vi "To CSV File.vi"(8 "error in (no error)":errorcluster, 9 "Path":path, 10 "engine configuration":refnum<class "engine configuration.lvclass">, 11 "module editor node in":refnum<class "module editor node.lvclass">) -> (0 "error out":errorcluster, 3 "module editor node out":refnum<class "module editor node.lvclass">)   [LabVIEW 2014, in "PL Framework Configuration Tool.lvlib" / "module editor node.lvclass"]
uses:
  module editor node.lvclass
  <vilib>/NI/Module Execution Interface/Engine Configuration/engine configuration.lvclass
  <vilib>/NI/Tag Bus Module Framework/module configuration/TBM module configuration.lvclass
  <vilib>/NI/Configuration Framework/serializable configuration/NISE_CEF_serializable configuration.lvclass
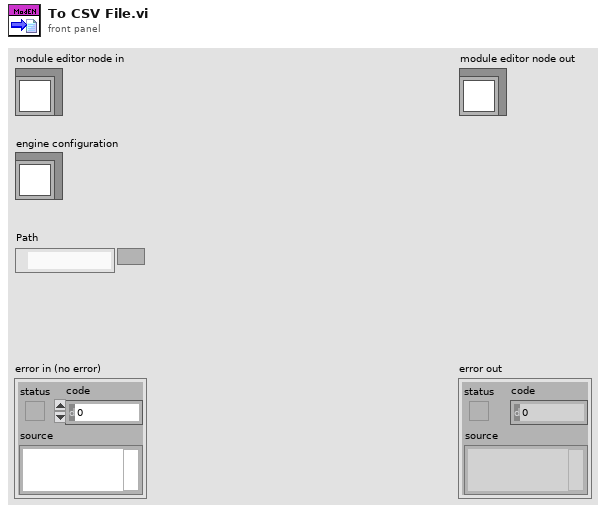
[diagram p1: front panel]
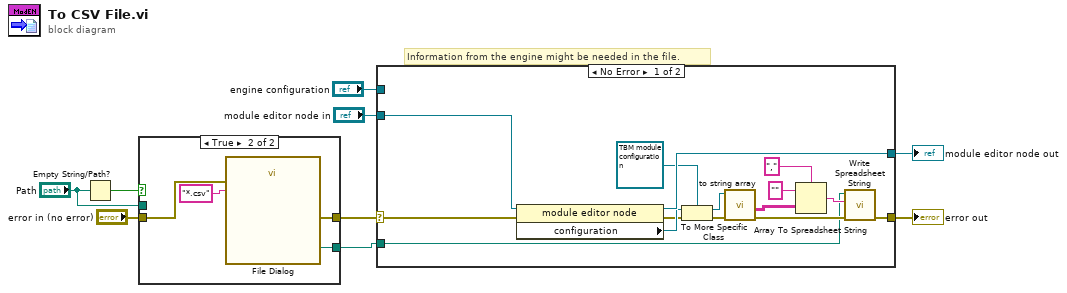
[diagram p0: block diagram]
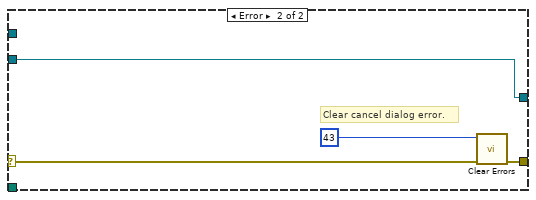
[diagram p3: hidden frame]
diagram:
  # "Information from the engine might be needed in the file."
  n1 = Empty String/Path?(string/path="Path") -> (empty?=w4:bool)
  n2 = case shown="True" w4 {
    tunnel: "error in (no error)" -> [w10 w14]
    tunnel: [w10 w13] -> w2
    tunnel: [w11 w12] -> w1
    tunnel: "Path" -> [w11 _]
    frame False {
    }
    frame True {
      n3 = call "File Dialog"("error in"=w14, "pattern (all files)"="*.csv") -> ("selected path"=w12:path, "error out"=w13:errorcluster)  [unwired: 10 in, 2 out]
    }
  }
  n4 = case shown="No Error" w2 {
    selector: w2 -> [w17 w33]
    tunnel: [w23 w32] -> w9
    tunnel: [w29 w34] -> w7
    tunnel: "module editor node in" -> [w30 w34]
    tunnel: "engine configuration" -> [_ _]
    tunnel: w1 -> [w16 _]
    frame No Error {
      n5 = property class="module editor node"(reference=w30, error in=w17) -> (reference out=w29:refnum<class "module editor node.lvclass">, error out=w18:errorcluster, "configuration"=w28:refnum<class "NISE_CEF_serializable configuration.lvclass">)
      n6 = To More Specific Class(target class=refnum<class "TBM module configuration.lvclass"> refnum ("module configuration in"), reference=w28, error in=w18) -> (specific class reference=w26:refnum<class "TBM module configuration.lvclass">, error out=w25:errorcluster)
      n7 = call-dynamic "to string array.vi"("error in (no error)"=w25, "module configuration in"=w26) -> ("error out"=w24:errorcluster, "Array"=w22:string[][])  [unwired: 6 in, 2 out]
      n8 = Array To Spreadsheet String(delimiter (Tab)=",", array=w22, 3:"" ("format string")) -> (spreadsheet string=w21:string)
      n9 = call <vilib>:"Write Spreadsheet String.vi"("error in"=w24, "spreadsheet string"=w21, "file path (dialog if empty)"=w16) -> ("error out"=w23:errorcluster)  [unwired: 7 in, 1 out]
    }
    frame Error {
      # "Clear cancel dialog error."
      n10 = call <vilib>:"Clear Errors.vi"("error in (no error)"=w33, "specific error code to clear (0: all)"=43) -> ("error out"=w32:errorcluster)  [unwired: 4 in, 1 out]
    }
  }
  "error out" <- w9
  "module editor node out" <- w7
